vi "例程30-公式波形VI的使用.vi"() -> ()   [LabVIEW 2016]
uses:
  <vilib>/measure/NI_MAPro.lvlib
panel:
  in  "停止":bool
  out "波形图":waveform(dbl)(graph)
  out "signal out":waveform(dbl) caption="信号输出"
  in  "sampling info":cluster{"Fs":dbl, "#s":dbl}={"Fs"=1000.0, "#s"=1000.0} caption="采样信息" {"Fs" format="%.2p"}
  in  "offset":dbl caption="偏移量" format="%0.2p"
  in  "reset signal":bool caption="重置信号"
  in  "formula":string="sin(w*t)*sin(2*pi(1)*t)" caption="公式"
  in  "amplitude":dbl=1.0 caption="幅值" format="%0.2p"
  in  "frequency":dbl=10.0 caption="频率" format="%0.2p"
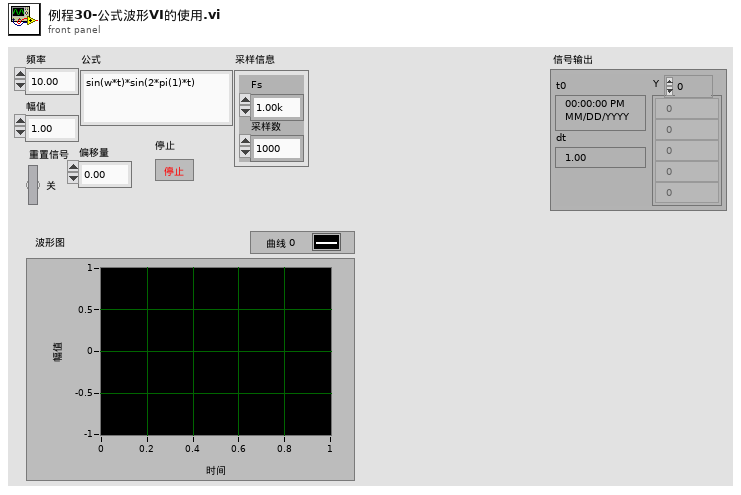
[diagram p1: front panel]
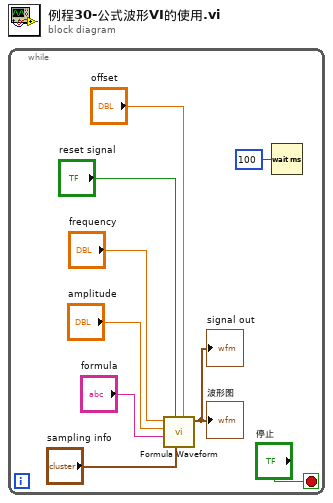
[diagram p0: block diagram]
diagram:
  n1 = while {
    stop <- "停止" stop-if-true
    n2 = call <vilib>:"Formula Waveform.vi"("offset"="offset", "sampling info"="sampling info", "reset signal"="reset signal", "formula"="formula", "amplitude"="amplitude", "frequency"="frequency") -> ("signal out"=→"signal out" →"波形图":waveform(dbl))  [unwired: 4 in, 1 out]
    n3 = Wait (ms)(milliseconds to wait=u32 100 ("等待时间（毫秒）")) -> ()  [unwired: 1 out]
  }
